vi "Initialize Instrument.vi"(8 "error in (no error)":errorcluster {"code" format="%.0x"}, 10 "Instr Resource Str":string, 11 "NI Switch.lvclass in":refnum<class "NI Switch.lvclass">) -> (0 "error out":errorcluster, 3 "NI Switch.lvclass out":refnum<class "NI Switch.lvclass">)   [LabVIEW 2011, in "NI Switch.lvclass"]
uses:
  NI Switch.lvclass
  <instrlib>/niSwitch/niSwitch.LLB/niSwitch Topologies.ctl
  NI Switch.lvclass/NI Switch.ctl
  <instrlib>/niSwitch/niSwitch.LLB/niSwitch Connect Channels (Single).vi
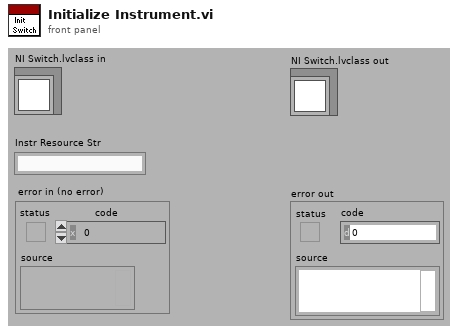
[diagram p1: front panel]
types:
  T1 = typedef "niSwitch Topologies.ctl" = string
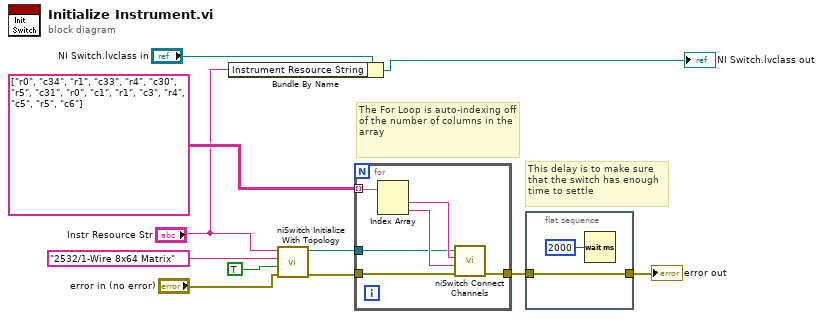
[diagram p0: block diagram]
diagram:
  # "This delay is to make sure that the switch has enough time to settle"
  # "The For Loop is auto-indexing off \nof the number of columns in the\narray"
  n1 = Bundle By Name(cluster="NI Switch.lvclass in", "Instrument Resource String"="Instr Resource Str") -> (→"NI Switch.lvclass out":refnum<class "NI Switch.lvclass">)
  n2 = call <instrlib>:"niSwitch Initialize With Topology.vi"("error in (no error)"="error in (no error)", "reset device (boolean value)"=TRUE ("reset device (Yes)"), "topology name"=T1 "2532/1-Wire 8x64 Matrix", "resource name"="Instr Resource Str") -> ("error out"=w9:errorcluster, "instrument handle out"=w10:refnum<k15>)  [unwired: 1 in, 5 out]
  n3 = for {
    tunnel: string[][] [["r0", "c34"], ["r1", "c33"], ["r4", "c30"], ["r5", "c31"], ["r0", "c1"], ["r1", "c3"], ["r4", "c5"], ["r5", "c6"]] -> [w17] mode=indexing
    tunnel: w10 -> [w14]
    tunnel: w9 -> [w13]
    tunnel: [w12] -> w5
    n4 = Index Array(array=w17) -> (element #1=w16:string, element #2=w15:string)  [unwired: 2 in]
    n5 = call-poly <instrlib>:"niSwitch Connect Channels.vi"("error in (no error)"=w13, "channel 2"=w15, "channel 1"=w16, "instrument handle"=w14) -> ("error out"=w12:errorcluster)  [unwired: 6 in, 1 out]
  }
  n6 = flat-sequence {
    tunnel: w5 -> [w19]
    tunnel: [w19] -> w4
    frame #0 {
      n7 = Wait (ms)(milliseconds to wait=u32 2000) -> ()  [unwired: 1 out]
    }
  }
  "error out" <- w4
